vi "S8300E_BP_BSPARE_WIH.vi"() -> ()   [LabVIEW 2011]
panel:
  out "prelog2":string
  out "FinalLog1":string
  out "LOG1":string
  out "Finallog2":string
  out "Test CMD":T1(array[cluster])
  out "Init CMD":T2(array[cluster])
  out "VISA Handle Array":refnum<visa-resource-name>[](array[refnum])
  out "VISA6":refnum<visa-resource-name>
  out "VISA9":refnum<visa-resource-name>
  out "BEGIN TIME":u32
  out "進行狀況":string
  # "2015-5-28"
  # "S8300E BackPlane  BSPARE"
  # "Error Code:BP-BSP"
  # "PC Com9 Baud  115200 -->S8300E MB\nPC COM6 Baud 115200 -->Test Board UART"
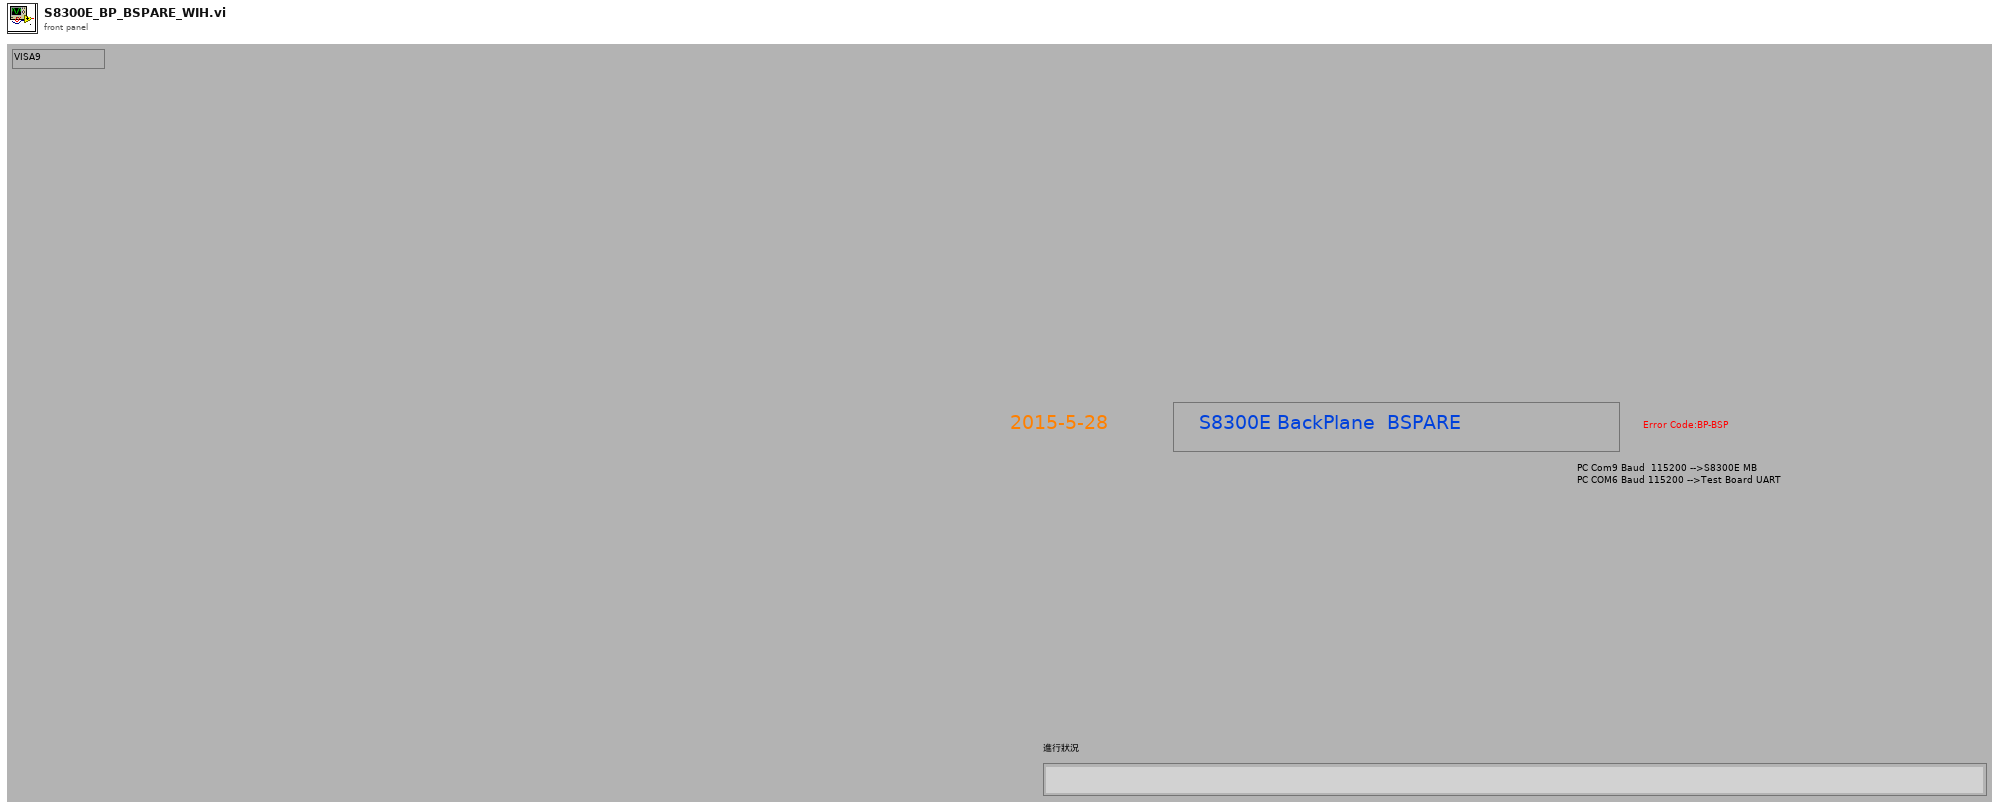
[diagram p1: front panel]
types:
  T1 = cluster{"VISA9":refnum<visa-resource-name>, "Find this String":string, "Find this String":string, "Find this String":string}[]
  T2 = cluster{"Find this String":string, "Find this String":string, "Find this String":string}[]
  T3 = cluster{string, "Find this String":string, "Find this String":string}
  T4 = cluster{"VISA6":refnum<visa-resource-name>, string, "Find this String":string, "Find this String":string}
  T5 = cluster{"VISA9":refnum<visa-resource-name>, string, "Find this String":string, "Find this String":string}
  T6 = cluster{string, "Find this String":string, "Find this String":string}[]
  T7 = cluster{"VISA9":refnum<visa-resource-name>, string, "Find this String":string, "Find this String":string}[]
  T8 = cluster{"Find this String":string, "Find this String":string, "Find this String":string}
  T9 = cluster{"VISA9":refnum<visa-resource-name>, "Find this String":string, "Find this String":string, "Find this String":string}
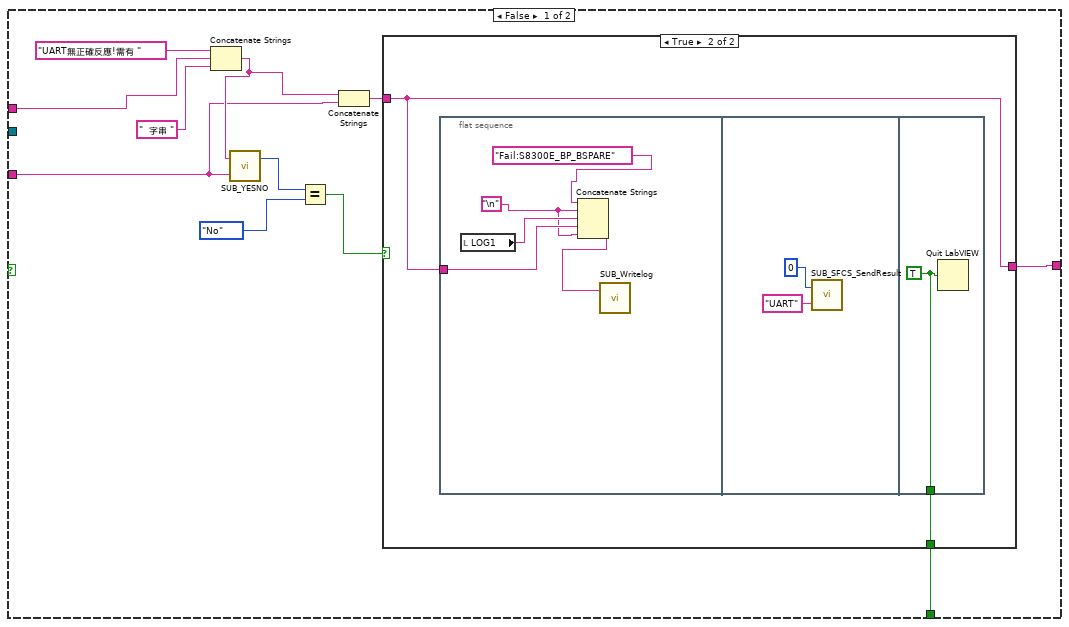
[diagram p3: hidden frame]
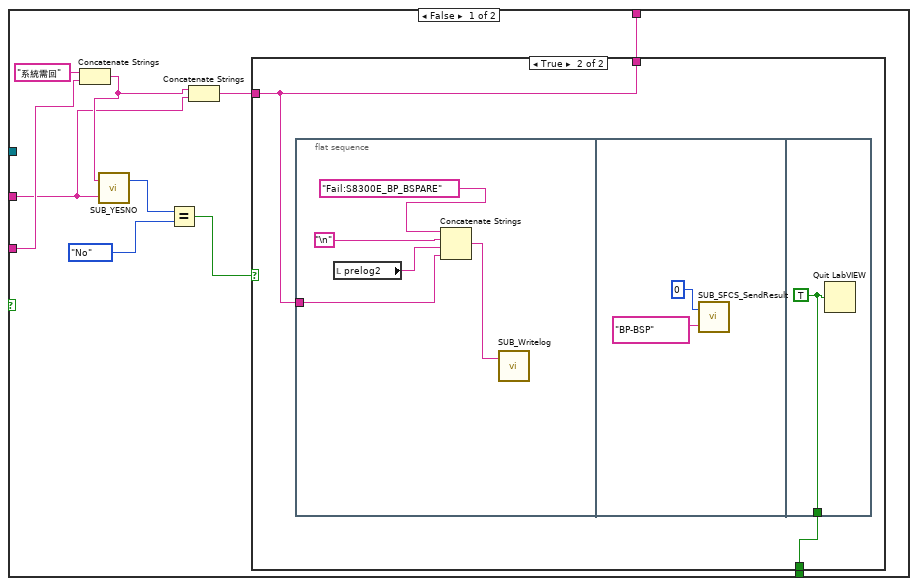
[diagram p5: hidden frame]
diagram:
  n1 = flat-sequence {
    tunnel: [w13] -> w2
    tunnel: w2 -> [w16]
    tunnel: [w90] -> w1
    tunnel: w1 -> [w91]
    frame #0 {
      n2 = Tick Count (ms)() -> (millisecond timer value=→"BEGIN TIME":u32)
    }
    frame #1 {
      n3 = Request Deallocation(TRUE ("flag")) -> ()
      n4 = property on="進行狀況" class="Str"("Blinking"=TRUE) -> ()  [unwired: 2 in, 2 out]
      "進行狀況" <- "進入測試準備中...." ("進行狀況")
    }
    frame #2 {
      n5 = call "SUB_SearchFile_inFolder.vi"("Search Filename in Folder"="S8300E_sfcs_misc.txt") -> ("File Existing True/Flase"=w7:bool)  [unwired: 1 in]
      n6 = case shown="False" w7 {
        frame False {
          n7 = flat-sequence {
            frame #0 {
              n8 = call "Display Message to User"() -> ()  [unwired: 10 in, 2 out]
            }
            frame #1 {
              n9 = call "SUB_Writelog.vi"("Pass/Fail"="Fail:S8300E_BP_BSPARE") -> ()  [unwired: 2 in]
            }
            frame #2 {
              n10 = Quit LabVIEW(quit? (T)=TRUE) -> ()
            }
          }
        }
        frame True {
        }
      }
    }
    frame #3 {
      n11 = call "SUB_COM1_CLOSE.vi"("VISA resource name"=refnum<visa-resource-name> "COM6") -> ()  [unwired: 3 in]
    }
    frame #4 {
      n12 = call "SUB_COM1_CLOSE.vi"("VISA resource name"=refnum<visa-resource-name> "COM9") -> ()  [unwired: 3 in]
    }
    frame #5 {
      n13 = call "SUB_COM_INIT.vi"("baud rate (9600)"=u32 115200, "VISA resource name"=refnum<visa-resource-name> "COM6") -> ("VISA resource name out"=w13:refnum<visa-resource-name>)  [unwired: 1 out]
      "VISA6" <- w13
    }
    frame #6 {
      n14 = call "SUB_COM9_INIT.vi"("baud rate"=u32 115200) -> ("VISA resource name out"=w18:refnum<visa-resource-name>)  [unwired: 1 in, 1 out]
      "VISA9" <- w18
      n15 = Build Array(w16, w18) -> (→"VISA Handle Array":refnum<visa-resource-name>[])
    }
    frame #7 {
      w20 = "\r"
      w21 = "PT1" ("Find this String")
      n16 = local read "VISA9"() -> (w31:refnum<visa-resource-name>)
      n17 = Concatenate Strings("PT2" ("Find this String"), "\r") -> (w22:string)
      n18 = local read "VISA6"() -> (w32:refnum<visa-resource-name>)
      n19 = Concatenate Strings(w21, w20, w21, w20) -> (w25:string)
      n20 = Concatenate Strings("./bac.sh -b", "\r") -> (w45:string)
      n21 = Concatenate Strings("./bac.sh -b", "\r") -> (w38:string)
      n22 = Bundle(w25, "Find this String"="PT1: Pass", "Find this String"="Checking COM6 Function...") -> (w35:T3)  [unwired: 1 in]
      n23 = Bundle("\r", "Find this String"="s8300e_func_test", "Find this String"="Checking COM9 Function") -> (w34:T3)  [unwired: 1 in]
      n24 = Bundle("VISA6"=w32, w25, "Find this String"="PT1: Pass", "Find this String"="G450 Output Signal Pattern1") -> (w30:T4)  [unwired: 1 in]
      n25 = Bundle("VISA9"=w31, w45, "Find this String"="PASSED=0x02", "Find this String"="Check G450 Pattern 1") -> (w29:T5)  [unwired: 1 in]
      n26 = Bundle("VISA6"=w32, w22, "Find this String"="PT2: Pass", "Find this String"="G450 Output Signal Pattern2") -> (w28:T4)  [unwired: 1 in]
      n27 = Bundle("VISA9"=w31, w38, "Find this String"="PASSED=0x01", "Find this String"="Check G450 Pattern 2") -> (w27:T5)  [unwired: 1 in]
      n28 = Build Array(w35, w34) -> (→"Init CMD":T6)
      n29 = Build Array(w30, w29, w28, w27) -> (→"Test CMD":T7)
    }
    frame #8 {
      n30 = while {
        shift-right: [w62] -> _
        shift-left: "" -> [w63]
        i -> [w67]
        stop <- w68 stop-if-true
        w61 = "Fail" ("Find this String")
        n31 = local read "VISA6"() -> (w56:refnum<visa-resource-name>)
        n32 = Greater Or Equal?(x=w67, y=3) -> (x >= y?=w65:bool)
        n33 = Tick Count (ms)() -> (millisecond timer value=w58:u32)
        n34 = call "SUB_WR_COM1_CbyCFindString_timeout.vi"("Begin time"=w58, "Find this String"=w61, "Timeout Seccond"=3.0, "cmd string"="\r", "duplicate VISA resource name 2"=w56) -> ("Output String"=w64:string, "Found String"=w60:bool)  [unwired: 2 out]
        n35 = Concatenate Strings(w63, w64) -> (w62:string)
        n36 = call "SUB_FindSpecificString.vi"("Find this String"=w61, "String data"=w62) -> ("Found"=w59:bool)  [unwired: 2 in, 1 out]
        n37 = Or(x=w60, y=w59) -> (x .or. y?=w57:bool)
        n38 = Or(x=w57, y=w65) -> (x .or. y?=w68:bool)
      }
    }
    frame #9 {
      n39 = local read "VISA6"() -> (w71:refnum<visa-resource-name>)
      n40 = call "SUB_COM_FLUSH_TXRX.vi"("VISA resource name"=w71) -> ()  [unwired: 2 in, 1 out]
    }
    frame #10 {
      n41 = while {
        shift-right: [w75] -> _
        shift-left: "" -> [w82]
        i -> [w76]
        stop <- w77 stop-if-true
        w74 = "PT1: Pass" ("Find this String")
        n42 = local read "VISA6"() -> (w86:refnum<visa-resource-name>)
        n43 = Tick Count (ms)() -> (millisecond timer value=w85:u32)
        n44 = Concatenate Strings("PT1" ("string"), "\r") -> (w87:string)
        n45 = call "SUB_WR_COM1_CbyCFindString_timeout.vi"("Begin time"=w85, "Find this String"=w74, "Timeout Seccond"=3.0, "cmd string"=w87, "duplicate VISA resource name 2"=w86) -> ("Output String"=w83:string, "Found String"=w73:bool)  [unwired: 2 out]
        n46 = Greater Or Equal?(x=w76, y=3) -> (x >= y?=w80:bool)
        n47 = Concatenate Strings(w82, w83) -> (w75:string)
        n48 = call "SUB_FindSpecificString.vi"("Find this String"=w74, "String data"=w75) -> ("Found"=w79:bool)  [unwired: 2 in, 1 out]
        n49 = Or(x=w73, y=w79) -> (x .or. y?=w78:bool)
        n50 = Or(x=w78, y=w80) -> (x .or. y?=w77:bool)
      }
    }
    frame #11 {
      n51 = Tick Count (ms)() -> (millisecond timer value=w90:u32)
    }
    frame #12 {
      n52 = while {
        shift-right: [w102] -> _
        shift-left: "" -> [w103]
        tunnel: w91 -> [w94]
        stop <- w100 stop-if-true
        n53 = local read "VISA9"() -> (w93:refnum<visa-resource-name>)
        n54 = call "SUB_COM1Wrt.vi"("VISA resource name"=w93, "write buffer"="\r") -> ("duplicate VISA resource name"=w106:refnum<visa-resource-name>)  [unwired: 1 in, 1 out]
        n55 = Tick Count (ms)() -> (millisecond timer value=w98:u32)
        n56 = Subtract(x=w98, y=w94) -> (x-y=w97:u32)
        n57 = Greater Or Equal?(x=w97, y=u32 5000) -> (x >= y?=w95:bool)
        n58 = call "SUB_ContinueCom1Read.vi"("Numeric"=1200, "duplicate VISA resource name 2"=w106) -> ("String"=w104:string)  [unwired: 1 in, 2 out]
        n59 = Concatenate Strings(w103, w104) -> (w102:string)
        n60 = call "SUB_FindSpecificString.vi"("Find this String"="S8300E", "String data"=w102) -> ("Found"=w99:bool)  [unwired: 2 in, 1 out]
        n61 = Or(x=w99, y=w95) -> (x .or. y?=w100:bool)
      }
    }
    frame #13 {
      n62 = local read "Init CMD"() -> (w109:T2)
      n63 = Array Size(array=w109) -> (size(s)=w108:i32)
      n64 = for {
        N: w108 -> [_]
        i -> [w114]
        n65 = local read "VISA Handle Array"() -> (w116:refnum<visa-resource-name>[])
        n66 = local read "Init CMD"() -> (w115:T2)
        n67 = Index Array(array=w116, index=w114) -> (element=w110:refnum<visa-resource-name>)
        n68 = Index Array(array=w115, index=w114) -> (element=w113:T8)
        n69 = while {
          tunnel: w113 -> [w131]
          shift-right: [w123] -> w111
          shift-left: "" -> [w121]
          tunnel: w110 -> [w118]
          stop <- w132 stop-if-true
          n70 = call "SUB_COM_FLUSH_TXRX.vi"("VISA resource name"=w118) -> ("VISA resource name out"=w117:refnum<visa-resource-name>)  [unwired: 2 in]
          n71 = Tick Count (ms)() -> (millisecond timer value=w128:u32)
          n72 = Unbundle(w131) -> ("Find this String"=w129:string, "Find this String"=w126:string, "Find this String"=w130:string)
          n73 = call "SUB_ContinueCom1Read.vi"("Numeric"=9600, "duplicate VISA resource name 2"=w117) -> ("duplicate VISA resource name"=w119:refnum<visa-resource-name>)  [unwired: 1 in, 2 out]
          n74 = call "SUB_WR_COM1_CbyCFindString_timeout.vi"("Begin time"=w128, "Find this String"=w126, "Timeout Seccond"=5.0, "cmd string"=w129, "duplicate VISA resource name 2"=w119) -> ("Output String"=w125:string, "Found String"=w124:bool)  [unwired: 2 out]
          n75 = local write "進行狀況"(w130) -> ()
          n76 = case shown="True" w124 {
            tunnel: [w140 TRUE] -> w132
            tunnel: w126 -> [w138 _]
            tunnel: w125 -> [w135 w157]
            tunnel: [w134 w157] -> w122
            tunnel: w119 -> [_ w155]
            frame False {
              n77 = Concatenate Strings("UART無正確反應!需有 " ("Status"), w138, "  字串 " ("Status")) -> (w136:string)
              n78 = call "SUB_YESNO.vi"("Debug View"=w135, "Status"=w136) -> ("yes/no"=w143:enum32{"No Selection", "Yes", "No", "None"})  [unwired: 1 in]
              n79 = Equal?(x=w143, y=enum32{"No Selection", "Yes", "No", "None"}."No") -> (x = y?=w141:bool)
              n80 = Concatenate Strings(w136, w135) -> (w133:string)
              n81 = case shown="True" w141 {
                tunnel: [_ w146] -> w140
                tunnel: [w144 w145] -> w134
                tunnel: w133 -> [w144 w145]
                frame False {
                }
                frame True {
                  n82 = flat-sequence {
                    tunnel: w145 -> [w149]
                    tunnel: [w154] -> w146
                    frame #0 {
                      w148 = "\n"
                      n83 = local read "LOG1"() -> (w150:string)
                      n84 = Concatenate Strings("Fail:S8300E_BP_BSPARE" ("Pass/Fail"), w148, w150, w149, w148) -> (w147:string)
                      n85 = call "SUB_Writelog.vi"("Pass/Fail"=w147) -> ()  [unwired: 2 in]
                    }
                    frame #1 {
                      n86 = call "SUB_SFCS_SendResult.vi"("ErrorCode"="UART", "PASS_Fail (1/0)"=i8 0) -> ()  [unwired: 1 out]
                    }
                    frame #2 {
                      w154 = TRUE ("quit? (T)")
                      n87 = Quit LabVIEW(quit? (T)=w154) -> ()
                    }
                  }
                }
              }
            }
            frame True {
              n88 = call "SUB_ContinueCom1Read.vi"("Numeric"=9600, "duplicate VISA resource name 2"=w155) -> ()  [unwired: 1 in, 3 out]
            }
          }
          n89 = Concatenate Strings(w121, w122) -> (w123:string)
          "LOG1" <- w123
        }
        "FinalLog1" <- w111
      }
    }
    frame #14 {
      n90 = local read "VISA9"() -> (w161:refnum<visa-resource-name>)
      n91 = call "SUB_COM1Wrt.vi"("VISA resource name"=w161, "write buffer"="\r") -> ("duplicate VISA resource name"=w160:refnum<visa-resource-name>)  [unwired: 1 in, 1 out]
      n92 = call "SUB_ContinueCom1Read.vi"("Numeric"=9600, "duplicate VISA resource name 2"=w160) -> ()  [unwired: 1 in, 3 out]
    }
    frame #15 {
      n93 = local read "VISA6"() -> (w163:refnum<visa-resource-name>)
      n94 = call "SUB_COM1Wrt.vi"("VISA resource name"=w163, "write buffer"="\r") -> ("duplicate VISA resource name"=w164:refnum<visa-resource-name>)  [unwired: 1 in, 1 out]
      n95 = call "SUB_ContinueCom1Read.vi"("Numeric"=9600, "duplicate VISA resource name 2"=w164) -> ()  [unwired: 1 in, 3 out]
    }
    frame #16 {
      n96 = local read "Test CMD"() -> (w170:T1)
      n97 = Array Size(array=w170) -> (size(s)=w169:i32)
      n98 = for {
        N: w169 -> [_]
        shift-right: [w172] -> w167
        shift-left: "" -> [w171]
        i -> [w174]
        n99 = while {
          tunnel: w174 -> [w189]
          tunnel: [w185] -> w173
          stop <- w186 stop-if-true
          n100 = local read "Test CMD"() -> (w190:T1)
          n101 = Index Array(array=w190, index=w189) -> (element=w188:T9)
          n102 = Unbundle(w188) -> ("VISA9"=w177:refnum<visa-resource-name>, "Find this String"=w182:string, "Find this String"=w181:string, "Find this String"=w187:string)
          n103 = call "SUB_ContinueCom1Read.vi"("Numeric"=9600, "duplicate VISA resource name 2"=w177) -> ("duplicate VISA resource name"=w175:refnum<visa-resource-name>)  [unwired: 1 in, 2 out]
          n104 = Tick Count (ms)() -> (millisecond timer value=w183:u32)
          n105 = local write "進行狀況"(w187) -> ()
          n106 = call "SUB_WR_COM1_CbyCFindString_timeout.vi"("Begin time"=w183, "Find this String"=w181, "Timeout Seccond"=8.0, "cmd string"=w182, "duplicate VISA resource name 2"=w175) -> ("Output String"=w179:string, "Found String"=w180:bool)  [unwired: 2 out]
          n107 = Wait (ms)(milliseconds to wait=u32 100) -> ()  [unwired: 1 out]
          n108 = case shown="True" w180 {
            tunnel: w181 -> [w196 w216]
            tunnel: [w195 TRUE] -> w186
            tunnel: [w192 w214] -> w185
            tunnel: w179 -> [w193 _]
            tunnel: w175 -> [_ w212]
            frame False {
              n109 = Concatenate Strings("系統需回" ("string"), w196) -> (w194:string)
              n110 = call "SUB_YESNO.vi"("Debug View"=w193, "Status"=w194) -> ("yes/no"=w200:enum32{"No Selection", "Yes", "No", "None"})  [unwired: 1 in]
              n111 = Equal?(x=w200, y=enum32{"No Selection", "Yes", "No", "None"}."No") -> (x = y?=w198:bool)
              n112 = Concatenate Strings(w194, w193) -> (w191:string)
              n113 = case shown="True" w198 {
                tunnel: [_ w203] -> w195
                tunnel: [w201 w202] -> w192
                tunnel: w191 -> [w201 w202]
                frame False {
                }
                frame True {
                  n114 = flat-sequence {
                    tunnel: w202 -> [w204]
                    tunnel: [w211] -> w203
                    frame #0 {
                      n115 = local read "prelog2"() -> (w206:string)
                      n116 = Concatenate Strings("Fail:S8300E_BP_BSPARE" ("Pass/Fail"), "\n", w206, w204) -> (w205:string)
                      n117 = call "SUB_Writelog.vi"("Pass/Fail"=w205) -> ()  [unwired: 2 in]
                    }
                    frame #1 {
                      n118 = call "SUB_SFCS_SendResult.vi"("ErrorCode"="BP-BSP", "PASS_Fail (1/0)"=i8 0) -> ()  [unwired: 1 out]
                    }
                    frame #2 {
                      w211 = TRUE ("quit? (T)")
                      n119 = Quit LabVIEW(quit? (T)=w211) -> ()
                    }
                  }
                }
              }
            }
            frame True {
              n120 = Concatenate Strings(w216, "\r") -> (w214:string)
              n121 = call "SUB_ContinueCom1Read.vi"("Numeric"=9600, "duplicate VISA resource name 2"=w212) -> ()  [unwired: 1 in, 3 out]
            }
          }
        }
        n122 = Concatenate Strings(w171, w173) -> (w172:string)
        "prelog2" <- w172
      }
      "Finallog2" <- w167
    }
    frame #17 {
      n123 = call "SUB_COM1_CLOSE.vi"("VISA resource name"=refnum<visa-resource-name> "COM9") -> ()  [unwired: 3 in]
    }
    frame #18 {
      n124 = call "SUB_COM1_CLOSE.vi"("VISA resource name"=refnum<visa-resource-name> "COM6") -> ()  [unwired: 3 in]
    }
    frame #19 {
      w222 = "***Not Good ***" ("replace string (\"\")")
      w227 = "\n"
      n125 = local read "FinalLog1"() -> (w229:string)
      n126 = local read "Finallog2"() -> (w228:string)
      n127 = local read "BEGIN TIME"() -> (w232:u32)
      n128 = Tick Count (ms)() -> (millisecond timer value=w231:u32)
      n129 = call "SUB_CAL_TESTTIME.vi"("Test Item name"="S8300E_BP_BSPARE", "Stop tick time"=w231, "Start tick time"=w232) -> ("Test Time output"=w226:string)  [unwired: 2 in]
      n130 = Concatenate Strings("Pass:S8300E_BP_BSPARE", w227, w229, w227, w228, w227, w226) -> (w221:string)
      n131 = call "SUB_SEARCH_REPLACE_STR.vi"("replace string (\"\")"=w222, "search string"="FAILED", "input string"=w221) -> ("result string"=w224:string)  [unwired: 2 in]
      n132 = call "SUB_SEARCH_REPLACE_STR.vi"("replace string (\"\")"=w222, "search string"="FAIL", "input string"=w224) -> ("result string"=w220:string)  [unwired: 2 in]
      n133 = call "SUB_Writelog.vi"("Pass/Fail"=w220) -> ()  [unwired: 2 in]
    }
    frame #20 {
      n134 = Quit LabVIEW(quit? (T)=TRUE ("stop? (T)")) -> ()
    }
  }
